vi "Open.vi"(8 "error in (no error)":errorcluster, 10 "address":string, 11 "Instrument in":refnum<class "Instrument.lvclass">) -> (0 "error out":errorcluster, 3 "Instrument out":refnum<class "Instrument.lvclass">)   [LabVIEW 2019, in "Instrument.lvclass"]
uses:
  Instrument.lvclass
  Instrument.lvclass/Instrument.ctl
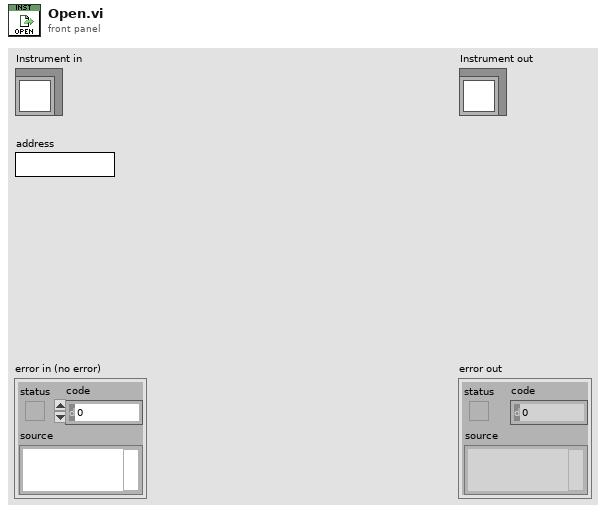
[diagram p1: front panel]
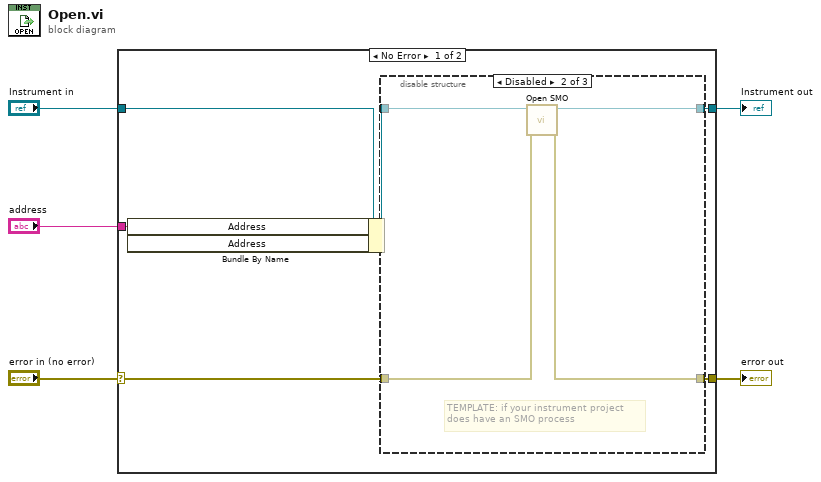
[diagram p0: block diagram]
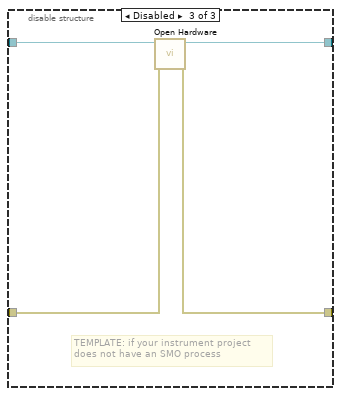
[diagram p3: hidden frame]
diagram:
  n1 = case shown="No Error" "error in (no error)" {
    selector: "error in (no error)" -> [w10 w23]
    tunnel: [w8 w23] -> w4
    tunnel: [w9 w22] -> w2
    tunnel: "Instrument in" -> [w11 w22]
    tunnel: "address" -> [w6 _]
    frame No Error {
      n2 = Bundle By Name(cluster=w11, "Address"=w6, "Address"=w6) -> (w7:refnum<class "Instrument.lvclass">)
      n3 = disable-structure shown="Disabled" {
        disable-tunnel: w7 -> [w13 w17 w18]
        disable-tunnel: w10 -> [w12 w15 w20]
        disable-tunnel: [w13 w16 w21] -> w9
        disable-tunnel: [w12 w14 w19] -> w8
        frame Enabled {
        }
        frame Disabled {
          # "TEMPLATE: if your instrument project\ndoes have an SMO process"
          n4 = call "Open SMO.vi"("error in (no error)"=w15, "Instrument in"=w17) -> ("error out"=w14:errorcluster, "Instrument out"=w16:refnum<class "Instrument.lvclass">)  [unwired: 8 in]
        }
        frame Disabled {
          # "TEMPLATE: if your instrument project\ndoes not have an SMO process"
          n5 = call-dynamic "Open Hardware.vi"("error in (no error)"=w20, "Instrument in"=w18) -> ("error out"=w19:errorcluster, "Instrument out"=w21:refnum<class "Instrument.lvclass">)  [unwired: 8 in]
        }
      }
    }
    frame Error {
    }
  }
  "error out" <- w4
  "Instrument out" <- w2
